vi "Page_AddRequirements.vi"(8 "error in (no error)":errorcluster, 11 "Configuration Paths":T1) -> (0 "error out":errorcluster, 3 "Configuration Paths out":T1)   [LabVIEW 2010]
uses:
  Config cluster.ctl
panel:
  in  "Delete":bool
  in  "Linked Requirements":i32(listbox)
  in  "Link to Req":bool
  out "Tree Element":string
  in  "Cancel Button":bool
  in  "OK Button":bool
  in  "Requirements":i32[](listbox)
  # "Available Requirements"
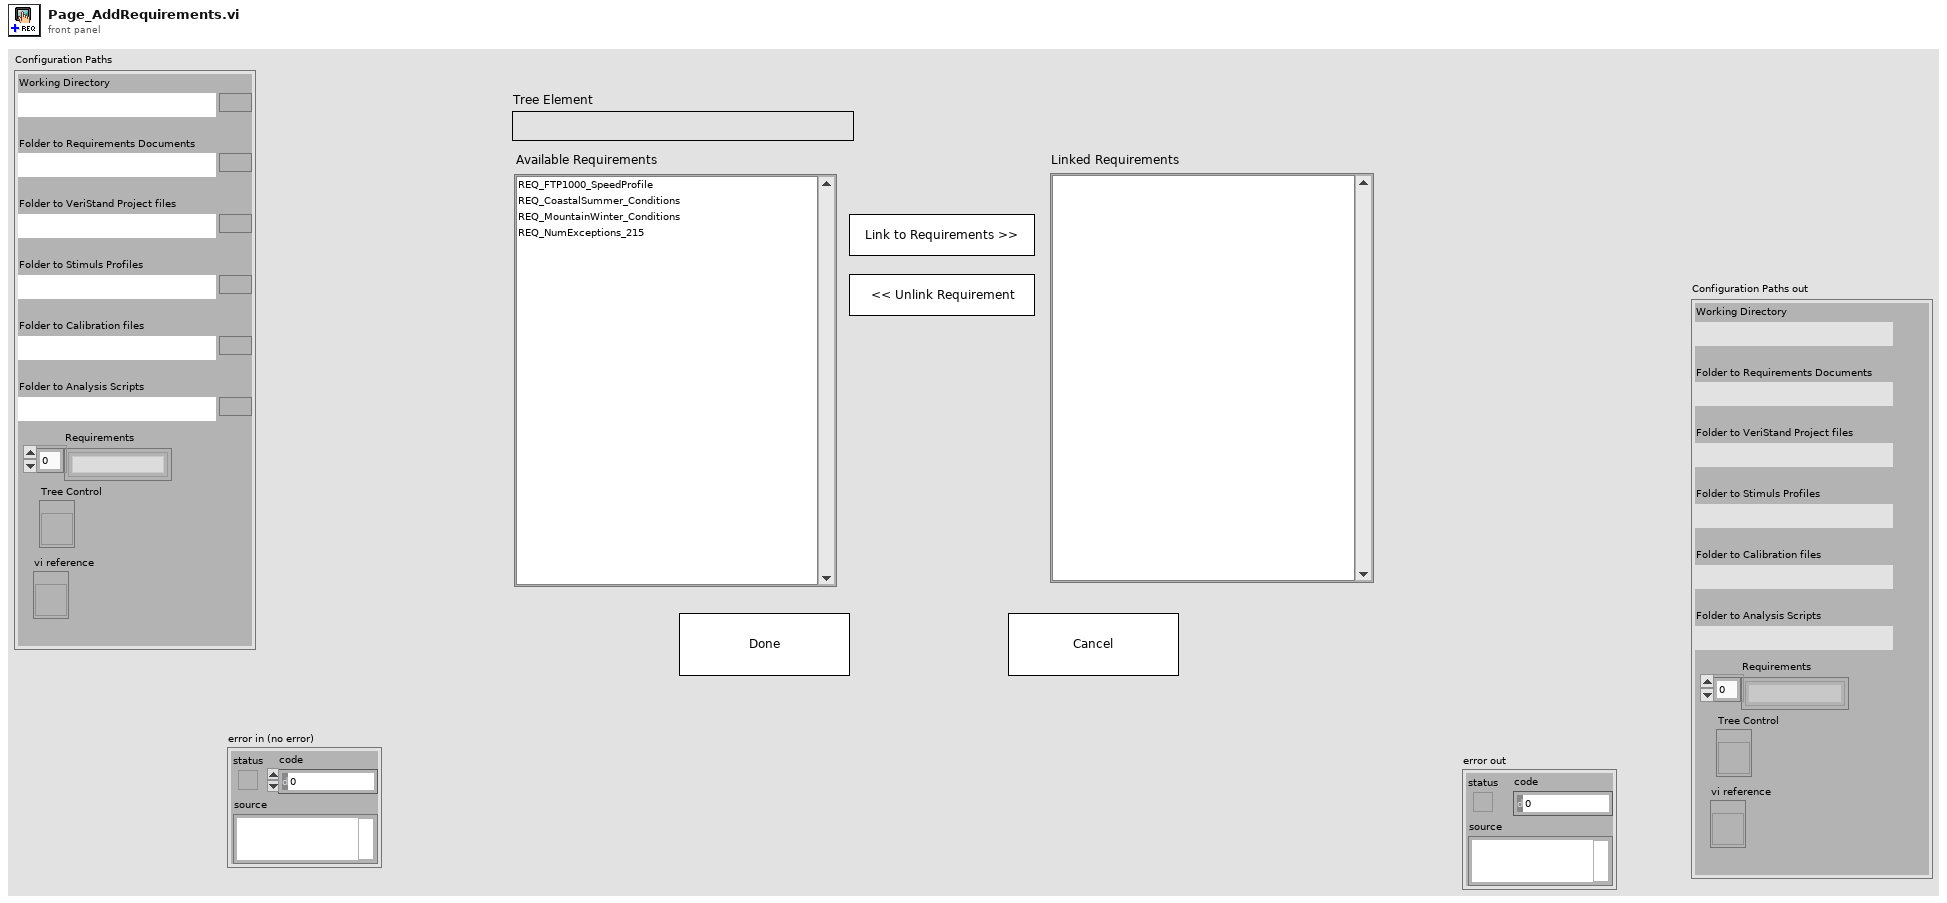
[diagram p1: front panel]
types:
  T1 = typedef "Config cluster.ctl" = cluster{"Working Directory":path, "Folder to Requirements Documents":path, "Folder to VeriStand Project files":path, "Folder to Stimuls Profiles":path, "Folder to Calibration files":path, "Folder to Analysis Scripts":path, "Requirements":string[], "Tree Control":refnum<vi>, "vi reference":refnum<vi>}
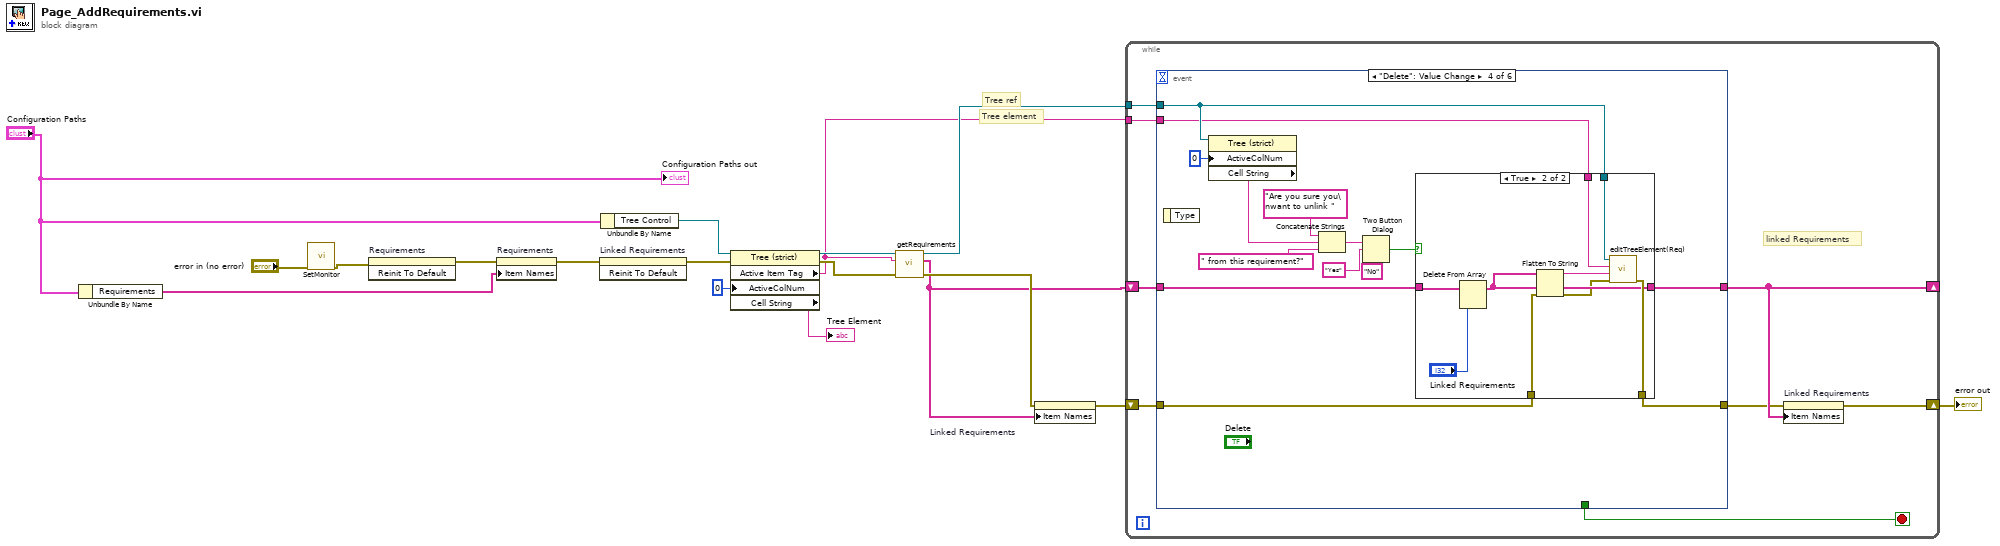
[diagram p0: block diagram]
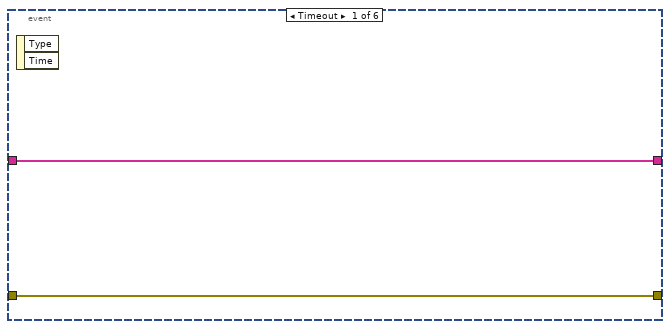
[diagram p2: hidden frame]
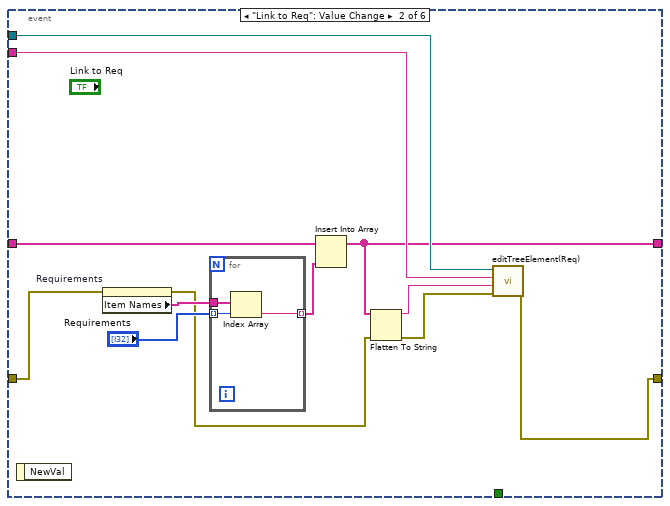
[diagram p3: hidden frame]
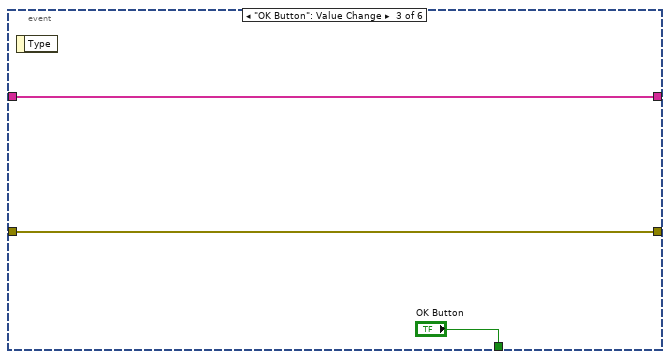
[diagram p4: hidden frame]
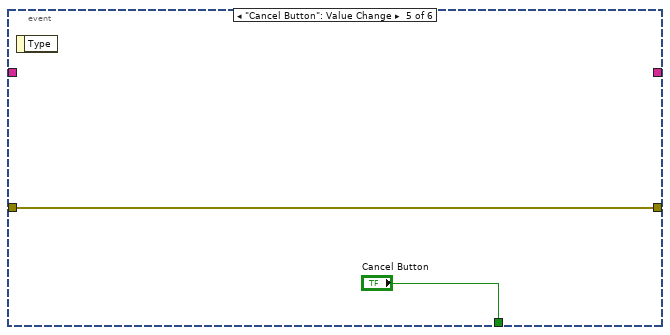
[diagram p6: hidden frame]
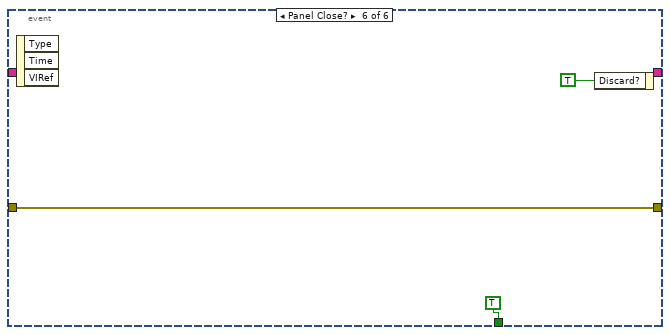
[diagram p7: hidden frame]
diagram:
  # "Tree element"
  # "Tree ref"
  n1 = Unbundle By Name("Configuration Paths") -> ("Requirements"=w11:string[])
  n2 = call "SetMonitor.vi"("error in (no error)"="error in (no error)") -> ("error out"=w2:errorcluster)  [unwired: 9 in, 1 out]
  n3 = invoke on="Requirements" class="LstBox (strict)" method="Reinit To Default"(error in=w2) -> (error out=w15:errorcluster)  [unwired: 2 in, 2 out]
  n4 = property on="Requirements" class="LstBox (strict)"(error in=w15, "Item Names"=w11) -> (error out=w13:errorcluster)  [unwired: 1 in, 1 out]
  n5 = invoke on="Linked Requirements" class="LstBox (strict)" method="Reinit To Default"(error in=w13) -> (error out=w12:errorcluster)  [unwired: 2 in, 2 out]
  n6 = Unbundle By Name("Configuration Paths") -> ("Tree Control"=w16:refnum<vi>)
  n7 = property class="Tree (strict)"(reference=w16, error in=w12, "ActiveColNum"=0 ("Active Cell:Active Column Number")) -> (reference out=w8:refnum<vi>, error out=w7:errorcluster, "Active Item Tag"=w4:string, "Cell String"=→"Tree Element":string)
  n8 = call "getRequirements.vi"("error in (no error)"=w7, "Active Item:Tag"=w4, "Tree Control"=w8) -> ("error out"=w6:errorcluster, "Requirements"=w3:string[], "Tree Control out"=w5:refnum<vi>)  [unwired: 6 in]
  n9 = property on="Linked Requirements" class="LstBox (strict)"(error in=w6, "Item Names"=w3) -> (error out=w18:errorcluster)  [unwired: 1 in, 1 out]
  n10 = while {
    tunnel: w5 -> [w25]
    tunnel: w4 -> [w24]
    shift-right: [w19] -> w17
    shift-left: w18 -> [w23]
    shift-right: [w22] -> _
    shift-left: w3 -> [w21]
    stop <- w26 stop-if-true
    # "linked Requirements"
    n11 = event shown="[3] \"Delete\": Value Change" {
      selector: _ -> [_ _ _ _ _ _]
      dyn-events: _ -> [_ _ _ _ _ _]
      timeout: _ -> [_ _ _ _ _ _]
      tunnel: [_ _ "OK Button" _ "Cancel Button" TRUE ("Cancel Button")] -> w26
      tunnel: w25 -> [_ w39 _ w52 _ _]
      tunnel: w24 -> [_ w38 _ w51 _ _]
      tunnel: w23 -> [w28 w31 w45 w47 w72 w76]
      tunnel: [w28 w36 w45 w50 w72 w76] -> w20
      tunnel: [w27 w32 w44 w48 _ _] -> w22
      tunnel: w21 -> [w27 w35 w44 w49 _ _]
      event Timeout {
        n12 = event-data() -> ()  [unwired: 1 in, 2 out]
      }
      event "Link to Req": Value Change {
        n13 = event-data() -> ()  [unwired: 1 in, 1 out]
        n14 = property on="Requirements" class="LstBox (strict)"(error in=w31) -> (error out=w29:errorcluster, "Item Names"=w40:string[])  [unwired: 1 in, 1 out]
        n15 = for {
          tunnel: w40 -> [w43]
          tunnel: [w42] -> w34 mode=indexing
          tunnel: "Requirements" -> [w41] mode=indexing
          n16 = Index Array(array=w43, index=w41) -> (element=w42:string)
        }
        n17 = Insert Into Array(array=w35, new element=w34) -> (w32:string[])  [unwired: 1 in]
        n18 = Flatten To String(anything=w32, error in (no error)=w29) -> (data string=w37:string, error out=w30:errorcluster)  [unwired: 2 in, 1 out]
        n19 = call "editTreeElement(Req).vi"("error in (no error)"=w30, "Req"=w37, "Active Item:Tag"=w38, "Tree Control in"=w39) -> ("error out"=w36:errorcluster)  [unwired: 7 in]
      }
      event "OK Button": Value Change {
        n20 = event-data() -> ()  [unwired: 1 in, 1 out]
      }
      event "Delete": Value Change {
        n21 = event-data() -> ()  [unwired: 1 in, 1 out]
        n22 = property class="Tree (strict)"(reference=w52, "ActiveColNum"=0 ("Active Cell:Active Column Number")) -> ("Cell String"=w56:string)  [unwired: 1 in, 2 out]
        n23 = Concatenate Strings("Are you sure you\nwant to unlink " ("message"), w56, " from this requirement?" ("string")) -> (w54:string)
        n24 = Two Button Dialog(message=w54, 1:"No" ("F button name (\"Cancel\")"), 2:"Yes" ("T button name (\"OK\")")) -> (T button?=w53:bool)
        n25 = case shown="True" w53 {
          tunnel: w52 -> [_ w70]
          tunnel: w51 -> [_ w69]
          tunnel: [w62 w68] -> w50
          tunnel: w49 -> [w61 w67]
          tunnel: [w61 w65] -> w48
          tunnel: w47 -> [w62 w64]
          frame False {
          }
          frame True {
            n26 = Delete From Array(array=w67, index="Linked Requirements") -> (array with subset deleted=w65:string[])  [unwired: 1 in, 1 out]
            n27 = Flatten To String(anything=w65, error in (no error)=w64) -> (data string=w71:string, error out=w63:errorcluster)  [unwired: 2 in, 1 out]
            n28 = call "editTreeElement(Req).vi"("error in (no error)"=w63, "Req"=w71, "Active Item:Tag"=w69, "Tree Control in"=w70) -> ("error out"=w68:errorcluster)  [unwired: 7 in]
          }
        }
      }
      event "Cancel Button": Value Change {
        n29 = event-data() -> ()  [unwired: 1 in, 1 out]
      }
      event Panel Close? {
        n30 = event-data() -> ()  [unwired: 1 in, 3 out]
        n31 = event-data("Discard?"=TRUE) -> ()  [unwired: 1 in, 1 out]
      }
    }
    n32 = property on="Linked Requirements" class="LstBox (strict)"(error in=w20, "Item Names"=w22) -> (error out=w19:errorcluster)  [unwired: 1 in, 1 out]
  }
  "error out" <- w17
  "Configuration Paths out" <- "Configuration Paths"
